vi "Validate hazard.vi"(9 "y":dbl, 10 "x":dbl) -> (3 "Valid":bool)   [LabVIEW 2015]
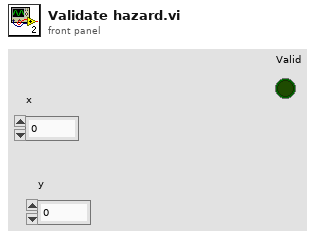
[diagram p1: front panel]
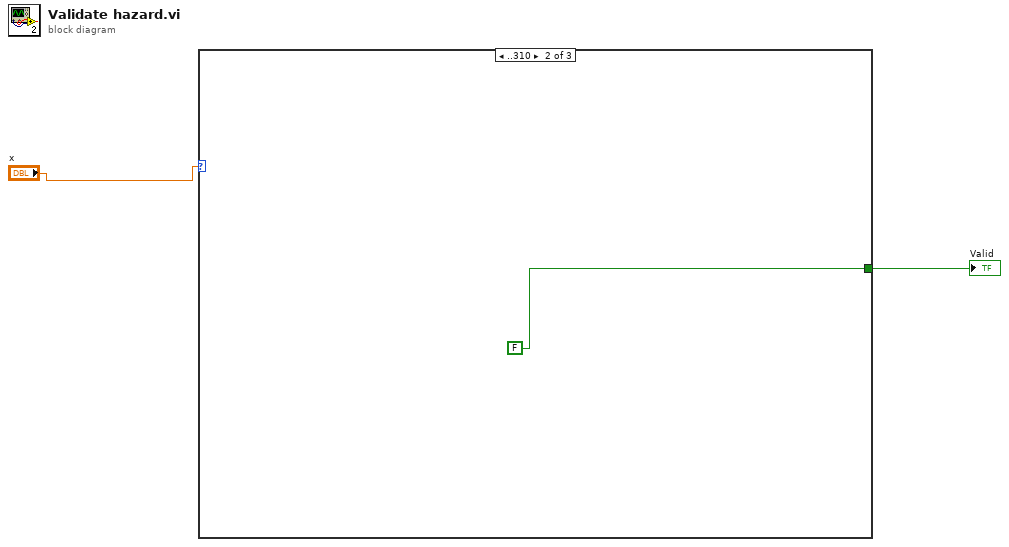
[diagram p0: block diagram]
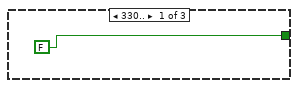
[diagram p2: hidden frame]
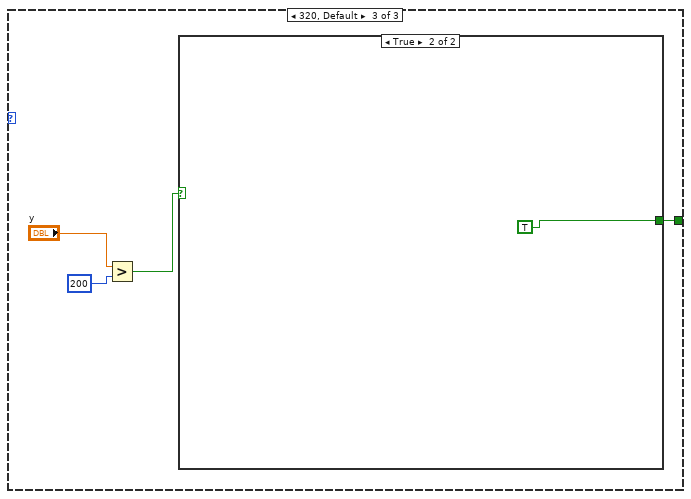
[diagram p3: hidden frame]
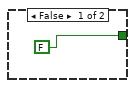
[diagram p4: hidden frame]
diagram:
  n1 = case shown="..310" "x" {
    tunnel: [FALSE FALSE w5] -> w2
    frame 330.. {
    }
    frame ..310 {
    }
    frame 320, Default {
      n2 = Greater?(x="y", y=200) -> (0:w6:bool)
      n3 = case shown="True" w6 {
        tunnel: [FALSE TRUE] -> w5
        frame False {
        }
        frame True {
        }
      }
    }
  }
  "Valid" <- w2
